vi "RVHR - Settings.vi"(7 "Initialise?":bool, 8 "error in (no error)":errorcluster) -> (0 "Error":errorcluster, 2 "Cancelled?":bool, 3 "Supervisory Config Cluster In":T4)   [LabVIEW 2024]
uses:
  Buttons/Select File.ctl
  Buttons/OK.ctl
  Buttons/Cancel.ctl
  Controls/RVHR - Reporting Settings.ctl
  Controls/RVHR - Setting refs.ctl
panel:
  in  "Image Distance (m)":dbl
  out "Settings":string
  in  "Select Button":T1 caption="Select"
  in  "OK Button":T2
  in  "Cancel Button":T3
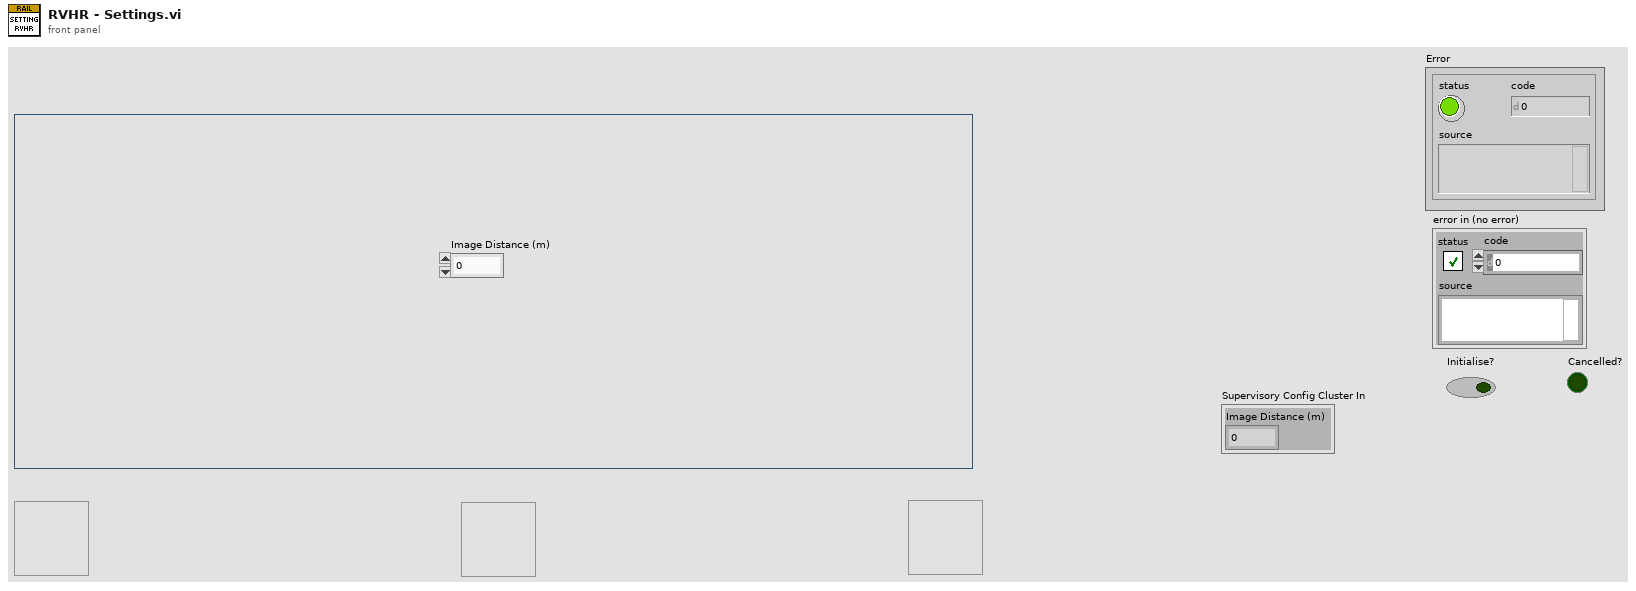
[diagram p1: front panel]
types:
  T1 = typedef "Select File.ctl" = bool
  T2 = typedef "OK.ctl" = bool
  T3 = typedef "Cancel.ctl" = bool
  T4 = typedef "RVHR - Reporting Settings.ctl" = cluster{"Image Distance (m)":dbl}
  T5 = typedef "RVHR - Setting refs.ctl" = cluster{"SETTING_1":refnum<vi>, "Settings":refnum<vi>}
  T6 = typedef "Supervisory Config Cluster.ctl" = cluster{"UI Information":T7, "Test Cluster":T12, "RV-HR Settings Cluster":T13}
  T7 = typedef "UI Init Config Info.ctl" = cluster{"Header Image":path, "Language":T8, "First Run?":bool, "Setup Camera?":bool, "Device Type":T9, "Encoder Type":T10, "Version":T11, "port":i32, "greyscale":bool, "camera index":i32}
  T8 = typedef "Language.ctl" = enum16{"English", "Chinese", "German"}
  T9 = typedef "Device_Type.ctl" = enum16{"CAT", "Bi-CAT", "YRCA", "RCA", "RV-HR", "TV-HR"}
  T10 = typedef "EncoderType.ctl" = enum16{"Tacho", "Quadrature"}
  T11 = typedef "Software Version.ctl" = enum16{"RailMeasurement_CAT", "RailMeasurement_Master", "RailMeasurement_RCA", "RailMeasurement_CAT-V", "RailMeasurement_RCA-V", "RailMeasurement_RV-HR"}
  T12 = typedef "Test Cluster.ctl" = cluster{"Operator":string, "Description":string, "Line":string, "Start Position":dbl, "Run Length":dbl, "Sensor A Position":dbl, "Rail Side":bool, "Distance Direction":bool, "Path":path, "Sensor B Position":dbl, "Visible Chart Distance":dbl, "Company":string, "Ref Profile":string}
  T13 = typedef "Settings Cluster.ctl" = cluster{"Sensor A Calibration":dbl, "Integrator Time":dbl, "Encoder Spacing":dbl, "Encoder Threshold":dbl, "Sampling Distance":T14, "Swap Direction?":bool, "Min Walking Speed":dbl, "Max Walking Speed":dbl, "Distance Format":T15, "Sensor B Calibration":dbl, "Tacho Pulses/Rev":dbl, "Wheel Diameter":dbl, "Max Short Roughness":dbl, "Max Long Roughness":dbl, "Measuring Interval":dbl, "Measuring Length":dbl, "Wavelengths":dbl[], "Device Resolution":T16, "Detect Change in Direction?":bool, "Save Images?":bool, "Image Frequency":T14, "Save Video?":bool, "Image Offset":dbl, "Start Position at 0m?":bool, "Live Corrug Est.?":bool, "Wavelength Corrug":u8, "Distance Corrug":u8, "Update Corrug":u8}
  T14 = typedef "Sampling DIstance.ctl" = u16
  T15 = typedef "Distance Units.ctl" = u16
  T16 = typedef "Device_Resolution.ctl" = u16
  T17 = typedef "Language Text Cluster.ctl" = cluster{"Home":string, "Test Setup":string, "Run Test":string, "Configure":string, "Hardware Viewer":string, "Review Test":string, "Report":string, "Exit":string, "Device Connected?":string, "Test in Progress?":string, "Simulate?":string, "Device Type 1":string, "Device Type 2":string, "Device Type 3":string, "Device Type 4":string, "Device Type 5":string, "Device Type 6":string, "Device Type 7":string, "Software Version":string, "Support":string, "Operator":string, "Test Description":string, "Line":string, "Test Folder Path":string, "Test Folder Path RCA":string, "Start Position":string, "Sensor Position":string, "Sensor A Position":string, "Sensor B Position":string, "Visible Chart Distance":string, "Rail Side":string, "Rail A Side":string, "Distance Direction":string, "Start":string, "Distance Travelled":string, "Current Position":string, "Stop Test":string, "Pause Test":string, "Displacement":string, "Position":string, "Sensor Calibration":string, "Sensor A Calibration":string, "Sensor B Calibration":string, "Encoder Spacing":string, "Sampling Distance":string, "Tacho Pulses/Rev":string, "Wheel Diameter":string, "Sampling Distances":string[], "Distance Unit":string, "Distance Units":string[], "Swap Direction":string, "Language":string, "Device Resolution":string, "Device Resolutions":string[], "Detect Change in Direction":string, "Save Config":string, "Encoder Data":string, "Sensor Data":string, "Sensor A Data":string, "Sensor B Data":string, "Voltage":string, "Time (m:s)":string, "Unit mm/s/V":string, "Unit mm":string, "Unit km":string, "Unit m":string, "Start Test Message":string, "Stop Test Message":string, "Exit Message":string, "File Exists Message":string, "File Path Invalid Message":string, "Combine Error":string, "Combine Success":string, "Roller Comp Error":string, "Test Folder Path (Live)":string, "Folder Error":string, "Enc Count":string, "Run Start":string, "Run End":string, "Date":string, "Train":string, "Location":string, "Notes":string, "Heading_1":string, "Heading_2":string, "Left Rail":string, "Right Rail":string, "Left Exclusions":string, "Right Exclusions":string, "Settings":string, "Wavelength Ranges":string, "Y-Axis Limits":string, "Exc Limits":string, "Other Settings":string, "Distance/Page":string, "Distance/Pages":string[], "Gridlines":string, "Report Tolerance":string, "Manual Cut":string, "Plot Colour":string, "Plot Colours":string[], "EN Standard":string, "RiL Standard":string, "Custom Standard":string, "Resolution":string, "Resolutions":string[], "Exceedence Header":string, "Distance (km)":string, "Left (%)":string, "Right (%)":string, "Page":string, "Align":string, "Main":string, "Comparison":string, "Offset":string, "From":string, "To":string, "Of":string, "File":string, "Load New":string, "Load Comparison":string, "Discard Comparison":string, "Print Current Page":string, "Print All Pages":string, "Print Exceedence Report":string, "Plot Main":string, "No Comparison Data to Align":string, "Run Load Error":string, "Report Load Error":string, "Cut":string, "Remove":string, "Config Settings Unsaved":string, "Acquisition Paused":string, "Please Select One Option Below":string, "RCA is Now Stationary":string, "Reporting Setting":string, "Main Abbreviated":string, "Comparison Abbreviated":string, "Exceedence Abbreviated":string, "Align Comparison":string, "Rail Corrugation Analyser Reporting":string, "Show Exc. % in Graph":string, "Evaluate Sections <100m":string, "Evaluate Sections <0.062mile":string, "Section Too Short for Evaluation":string, "Language Change Prompt":string, "Show All":string, "Sections_km":string, "Sections_mi":string, "Vision":string, "Vision Report":string, "Vision Display":string, "Vision Displays":string[], "Save Images":string, "Image Frequency":string, "Section":string, "Brightness":string, "Contrast":string, "Shadow":string, "Sharpened":string, "Apply to all Images":string, "Reset":string, "Are you sure":string, "Image Processing":string, "Save Video":string, "Image Offset":string, "Camera Mode":string, "Camera Modes":string[], "Copy Page":string, "Copy Graphs":string, "Camera Mode Change Prompt":string, "Camera_1 Missing":string, "Camera_2 Missing":string, "Cameras Missing":string, "Camera Setup":string, "Camera_1 Connection Error":string, "Camera_2 Connection Error":string, "Cameras Connection Error":string, "No GPS":string, "No Signal":string, "Camera_1 Connected":string, "Camera_1 Not Connected":string, "Camera_2 Connected":string, "Camera_2 Not Connected":string, "Start Position at 0m?":string, "Continue":string, "New Test, Same Direction":string, "New Test, Opposite Direction":string, "Stop and Save":string, "Live Corrug Estimate":string, "Wavelength Corrug":string, "Distance Corrug ":string, "Update Corrug":string, "Company":string, "Ref Profile ":string}
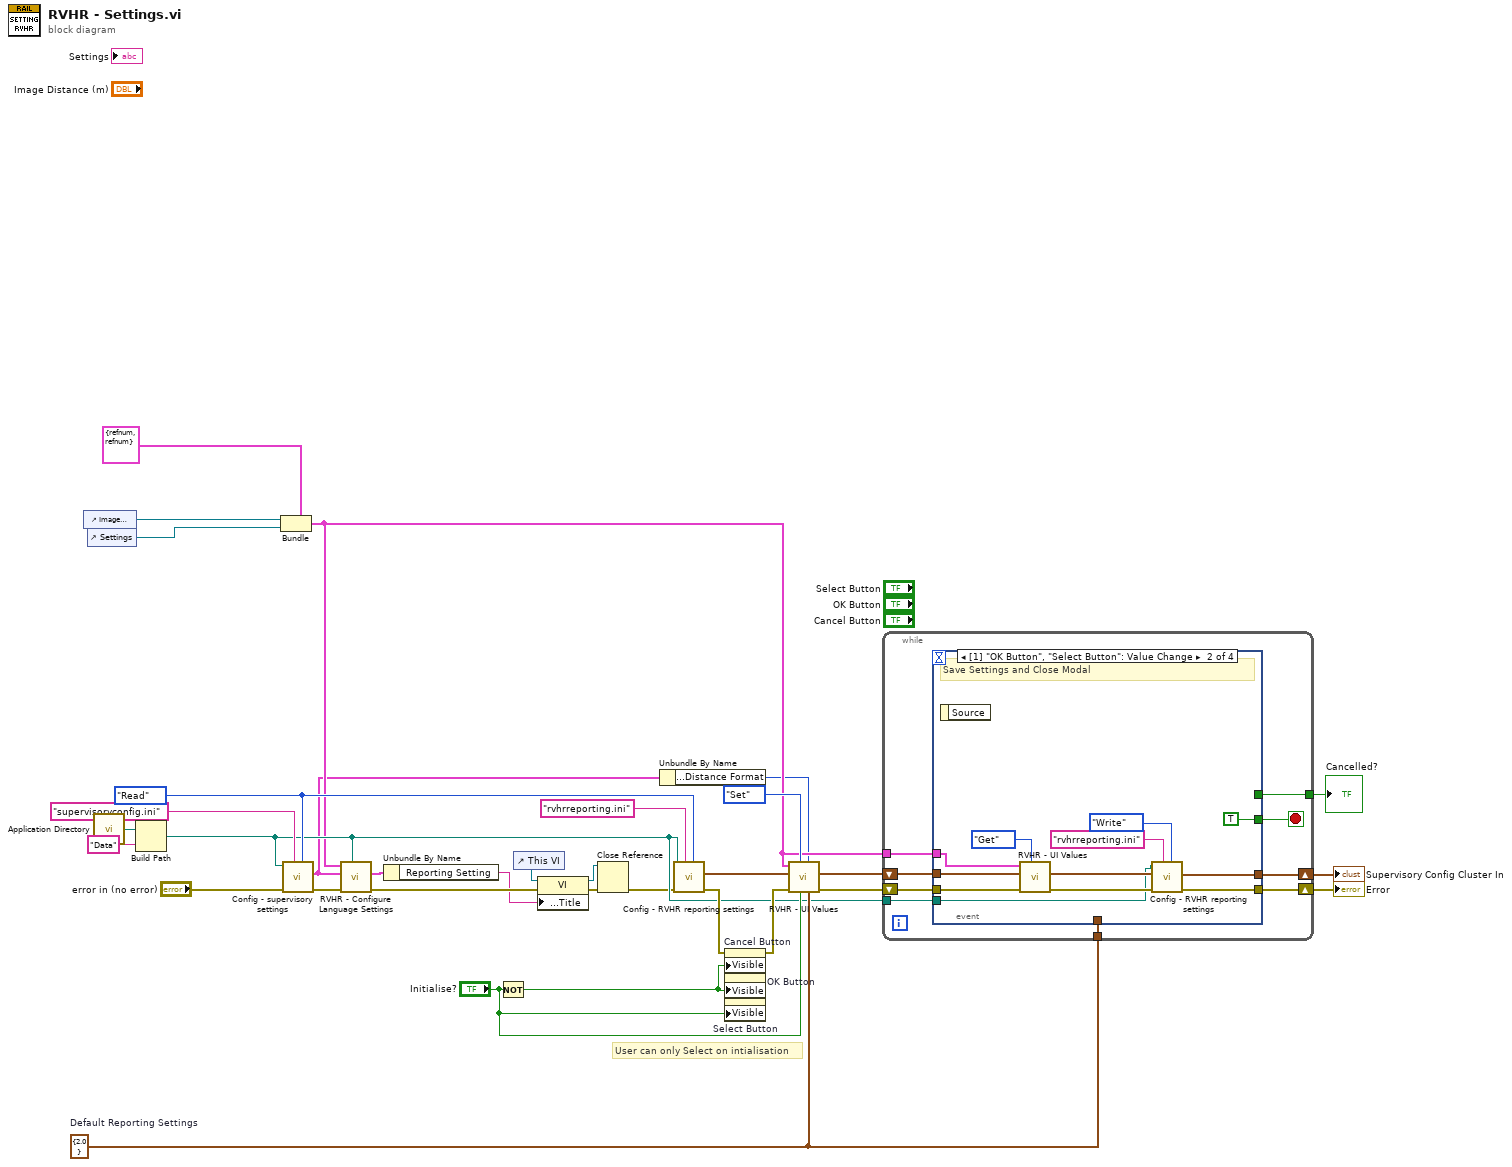
[diagram p0: block diagram]
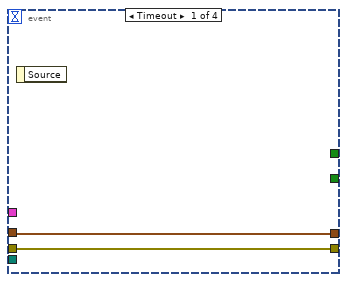
[diagram p2: hidden frame]
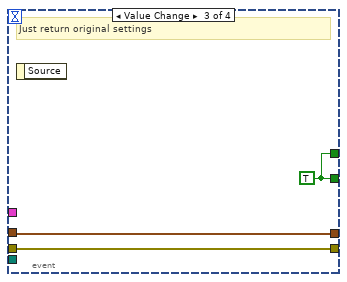
[diagram p3: hidden frame]
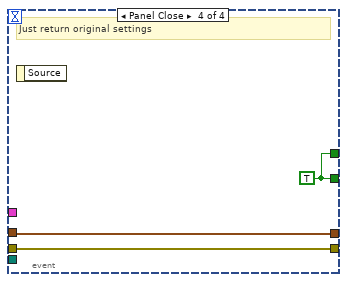
[diagram p4: hidden frame]
diagram:
  w22 = T4 {"Image Distance (m)"=2.0}  # Default Reporting Settings
  w18 = enum16{"Read", "Write"}."Read" (".ini Controller")
  # "User can only Select on intialisation"
  n1 = control-ref of="Image Distance (m)"() -> (w3:refnum<vi>)
  n2 = control-ref of="Settings"() -> (w11:refnum<vi>)
  n3 = call <vilib>:"Application Directory.vi"() -> ("Application Directory"=w1:path)
  n4 = Build Path(base path=w1, name or relative path="Data") -> (appended path=w15:path)
  n5 = Bundle(cluster=T5 {"SETTING_1"=refnum, "Settings"=refnum} ("output cluster"), "SETTING_1"=w3, "Settings"=w11) -> (w14:T5)
  n6 = call "Config - supervisory settings.vi"(".ini Controller"=w18, ".ini filename"="supervisoryconfig.ini", "error in (no error)"="error in (no error)", "Directory Path"=w15) -> ("error out"=w17:errorcluster, "Supervisory Config Cluster Out"=w13:T6)  [unwired: 5 in, 1 out]
  n7 = call "RVHR - Configure Language Settings.vi"("Directory Path"=w15, "error in (no error)"=w17, "Supervisory Config Cluster Out"=w13, "UI References"=w14) -> ("error out"=w10:errorcluster, "Language Config Cluster Out"=w5:T17)  [unwired: 6 in]
  n8 = Unbundle By Name(w5) -> ("Reporting Setting"=w4:string)
  n9 = Not(x="Initialise?") -> (.not. x?=w20:bool)
  n10 = control-ref of="This VI"() -> (w9:refnum<vi>)
  n11 = property class="VI"(reference=w9, error in=w10, "Front Panel.Title"=w4) -> (reference out=w7:refnum<vi>, error out=w8:errorcluster)
  n12 = Close Reference(reference=w7, error in (no error)=w8) -> (error out=w6:errorcluster)
  n13 = Unbundle By Name(w13) -> ("RV-HR Settings Cluster.Distance Format"=w12:T15)
  n14 = call "Config - RVHR reporting settings.vi"(".ini Controller"=w18, ".ini filename"="rvhrreporting.ini", "error in (no error)"=w6, "Directory Path"=w15) -> ("error out"=w24:errorcluster, "RVHR Config Cluster Out"=w28:T4)  [unwired: 5 in, 1 out]
  n15 = property on="Cancel Button" class="Bool"(error in=w24, "Visible"=w20) -> (error out=w23:errorcluster)  [unwired: 1 in, 1 out]
  n16 = property on="OK Button" class="Bool"("Visible"=w20) -> ()  [unwired: 2 in, 2 out]
  n17 = property on="Select Button" class="Bool"("Visible"="Initialise?") -> ()  [unwired: 2 in, 2 out]
  n18 = call "RVHR - UI Values.vi"("Default Reporting Settings"=w22, "Units"=w12, "Initialise?"="Initialise?", "Command"=enum16{"Set", "Get"}."Set", "error in (no error)"=w23, "Reporting IN"=w28, "UI Refs"=w14) -> ("error out"=w29:errorcluster, "Reporting Out"=w26:T4)  [unwired: 3 in]
  n19 = while {
    shift-right: [w39] -> w31
    shift-left: w26 -> [w38]
    shift-right: [w40] -> w30
    shift-left: w29 -> [w41]
    tunnel: w14 -> [w37]
    tunnel: w15 -> [w36]
    tunnel: [w35] -> w25
    tunnel: w22 -> [w34]
    stop <- w42 stop-if-true
    n20 = event shown="[1] \"OK Button\", \"Select Button\": Value Change" {
      selector: _ -> [_ _ _ _]
      dyn-events: _ -> [_ _ _ _]
      timeout: _ -> [_ _ _ _]
      tunnel: [_ TRUE ("Discard?") w57 w60] -> w42
      tunnel: w41 -> [w44 w53 w59 w62]
      tunnel: [w44 w56 w59 w62] -> w40
      tunnel: [w43 w55 w58 w61] -> w39
      tunnel: w38 -> [w43 w51 w58 w61]
      tunnel: w37 -> [_ w49 _ _]
      tunnel: w36 -> [_ w46 _ _]
      tunnel: [_ _ w57 w60] -> w35
      tunnel: w34 -> [_ _ _ _]
      event Timeout {
        n21 = event-data() -> ()  [unwired: 1 in, 1 out]
      }
      event Value Change {
        # "Save Settings and Close Modal"
        n22 = event-data() -> ()  [unwired: 1 in, 1 out]
        n23 = call "RVHR - UI Values.vi"("Command"=enum16{"Set", "Get"}."Get", "error in (no error)"=w53, "Reporting IN"=w51, "UI Refs"=w49) -> ("error out"=w52:errorcluster, "Reporting Out"=w50:T4)  [unwired: 6 in]
        n24 = call "Config - RVHR reporting settings.vi"(".ini Controller"=enum16{"Read", "Write"}."Write", ".ini filename"="rvhrreporting.ini", "error in (no error)"=w52, "RVHR Config Cluster In"=w50, "Directory Path"=w46) -> ("error out"=w56:errorcluster, "RVHR Config Cluster Out"=w55:T4)  [unwired: 4 in, 1 out]
      }
      event Value Change {
        w57 = TRUE ("Discard?")
        # "Just return original settings"
        n25 = event-data() -> ()  [unwired: 1 in, 1 out]
      }
      event Panel Close {
        w60 = TRUE ("Discard?")
        # "Just return original settings"
        n26 = event-data() -> ()  [unwired: 1 in, 1 out]
      }
    }
  }
  "Supervisory Config Cluster In" <- w31
  "Error" <- w30
  "Cancelled?" <- w25
